vi "Read Name.vi"(8 "error in (no error)":errorcluster, 11 "System in":refnum<class "System.lvclass">) -> (0 "error out":errorcluster, 2 "Name":string, 3 "System out":refnum<class "System.lvclass">)   [LabVIEW 2013, in "System.lvlib" / "System.lvclass"]
uses:
  System.lvclass
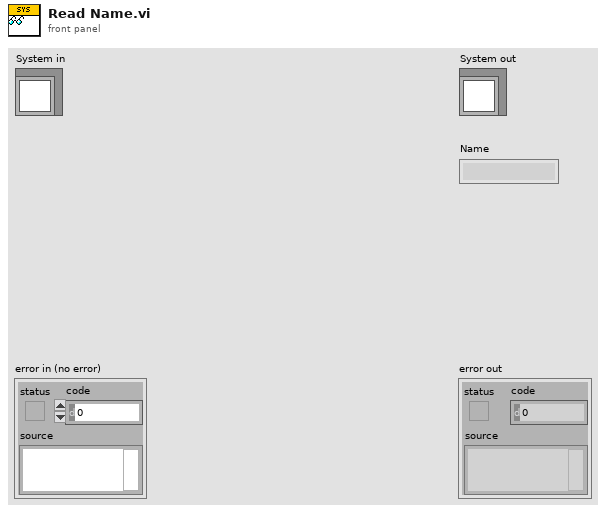
[diagram p1: front panel]
types:
  T1 = typedef "System.lvlib/System.lvclass/System Status.ctl" = cluster{"Current System State":T2, "System Health":enum16{"Unknown", "Good", "Poor", "Bad"}, "System Name":string, "Command Processor Status":T3}
  T2 = typedef "System.lvlib/System.lvclass/SystemStates.ctl" = enum16{"Unknown", "Running", "Stopped"}
  T3 = typedef "Command Processor.lvlib/Command Processor.lvclass/Command Processor Status.ctl" = cluster{"State Entry time":timestamp, "State Status":T4, "Command Processor Current State":string, "Command Status":T6}
  T4 = typedef "Current Previous State Status.ctl" = cluster{"Current State Status":T5, "Previous State Status":T5}
  T5 = typedef "State Status.ctl" = cluster{"State Name":string, "State Entry Time":timestamp, "State Exit Time":timestamp}
  T6 = typedef "Command Processor.lvlib/Command.lvlib/Command.lvclass/Command Status.ctl" = cluster{"Command Name":string, "Current State Status":T7, "Command Start Time":timestamp, "Command End Time":timestamp, "Previous State Status":T7}
  T7 = typedef "Command Processor.lvlib/Command.lvlib/Command.lvclass/State Status.ctl" = cluster{"State Name":string, "State Entry Time":timestamp, "State Exit Time":timestamp}
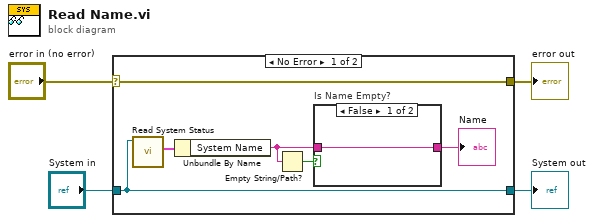
[diagram p0: block diagram]
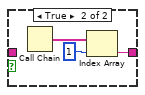
[diagram p2: hidden frame]
diagram:
  n1 = case shown="No Error" "error in (no error)" {
    selector: "error in (no error)" -> [w10 w15]
    tunnel: [w10 w15] -> w3
    tunnel: [w7 w16] -> w1
    tunnel: "System in" -> [w7 w16]
    frame No Error {
      n2 = call-dynamic "Read System Status.vi"("System in"=w7) -> ("System Status"=w6:T1)  [unwired: 8 in, 2 out]
      n3 = Unbundle By Name(w6) -> ("System Name"=w5:string)
      n4 = Empty String/Path?(string/path=w5) -> (empty?=w9:bool)
      n5 = case "Is Name Empty?" shown="False" w9 {
        tunnel: w5 -> [w11 _]
        tunnel: [w11 w12] -> w8
        frame False {
        }
        frame True {
          n6 = Call Chain() -> (call chain=w14:string[])
          n7 = Index Array(array=w14, index=1) -> (element=w12:string)
        }
      }
      "Name" <- w8
    }
    frame Error {
    }
  }
  "error out" <- w3
  "System out" <- w1
